vi "connection_process.vi"(6 "timeout (ms)":i32=1000, 11 "Connection":refnum<class "Connection.lvclass">) -> ()   [LabVIEW 2013, in "MQTT_Connection.lvlib" / "Connection.lvclass"]
uses:
  Connection.lvclass
  Connection.lvclass/Connection.ctl
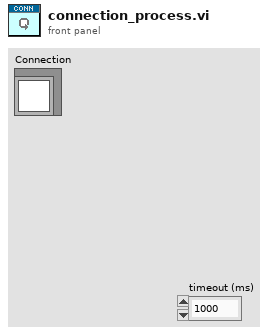
[diagram p1: front panel]
types:
  T1 = cluster{"Connection out":refnum<class "Connection.lvclass">, "error out":errorcluster}
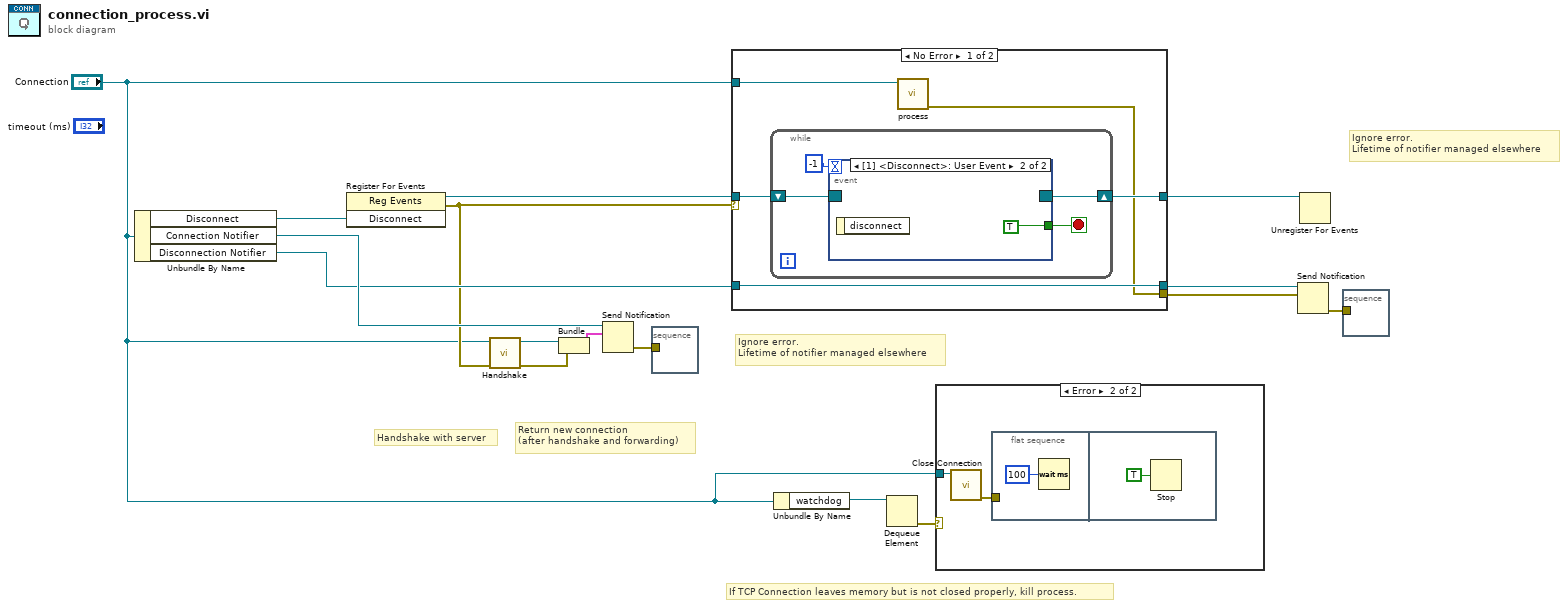
[diagram p0: block diagram]
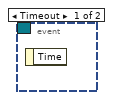
[diagram p3: hidden frame]
diagram:
  # "Return new connection\n(after handshake and forwarding)"
  # "Handshake with server"
  # "If TCP Connection leaves memory but is not closed properly, kill process."
  # "Ignore error.\nLifetime of notifier managed elsewhere"
  # "Ignore error.\nLifetime of notifier managed elsewhere"
  n1 = Unbundle By Name("Connection") -> ("Disconnect"=w13:refnum<user-event>, "Connection Notifier"=w12:refnum<notifier>, "Disconnection Notifier"=w9:refnum<notifier>)
  n2 = register-events(w13) -> (reference out=w14:refnum<event-registration>, error out=w6:errorcluster)  [unwired: 2 in]
  n3 = call-dynamic "Handshake.vi"("error in (no error)"=w6, "Connection in"="Connection") -> ("error out"=w5:errorcluster, "Connection out"=w3:refnum<class "Connection.lvclass">)  [unwired: 8 in]
  n4 = Bundle("Connection out"=w3, "error out"=w5) -> (w16:T1)  [unwired: 1 in]
  n5 = Send Notification(notification=w16, notifier=w12) -> (error out=w2:errorcluster)  [unwired: 1 in, 1 out]
  n6 = stacked-sequence {
    tunnel: w2 -> [_]
    frame #0 {
    }
  }
  n7 = case shown="No Error" w6 {
    selector: w6 -> [_ w28]
    tunnel: [w21 w29] -> w15
    tunnel: w14 -> [w20 w29]
    tunnel: [w17 w28] -> w11
    tunnel: w9 -> [w19 w27]
    tunnel: [w19 w27] -> w10
    tunnel: "Connection" -> [w18 _]
    frame No Error {
      n8 = while {
        shift-right: [w24] -> w21
        shift-left: w20 -> [w23]
        stop <- w22 stop-if-true
        n9 = event shown="[1] <Disconnect>: User Event" {
          selector: w23 -> [_ _]
          dyn-events: [_ _] -> w24
          timeout: -1 -> [_ _]
          tunnel: [_ TRUE] -> w22
          event Timeout {
            n10 = event-data() -> ()  [unwired: 1 in, 1 out]
          }
          event User Event {
            n11 = event-data() -> ()  [unwired: 1 in, 1 out]
          }
        }
      }
      n12 = call-dynamic "process.vi"("Connection in"=w18) -> ("error out"=w17:errorcluster)  [unwired: 9 in, 1 out]
    }
    frame Error {
    }
  }
  n13 = Unbundle By Name("Connection") -> ("watchdog"=w8:refnum<queue>)
  n14 = Dequeue Element(queue=w8) -> (error out=w7:errorcluster)  [unwired: 2 in, 3 out]
  n15 = case shown="Error" w7 {
    tunnel: "Connection" -> [_ w31]
    frame No Error {
    }
    frame Error {
      n16 = call "Close Connection.vi"("Connection in"=w31) -> ("error out"=w30:errorcluster)  [unwired: 9 in, 1 out]
      n17 = flat-sequence {
        tunnel: w30 -> [_]
        frame #0 {
          n18 = Wait (ms)(milliseconds to wait=u32 100) -> ()  [unwired: 1 out]
        }
        frame #1 {
          n19 = Stop(stop? (T)=TRUE) -> ()
        }
      }
    }
  }
  n20 = Send Notification(notification=w11, notifier=w10) -> (error out=w1:errorcluster)  [unwired: 1 in, 1 out]
  n21 = Unregister For Events(event registration refnum=w15) -> ()  [unwired: 1 in, 1 out]
  n22 = stacked-sequence {
    tunnel: w1 -> [_]
    frame #0 {
    }
  }
